vi "StatusTcpLink.vi"(0 "TCP Ref":refnum<k5>, 7 "VariableData":T1={"DecodeMode"="Stat", "LastSerial"=0, "NoReply"=FALSE, "StatCmd"="", "StatCmdReply"="", "StatCmdReplySerial"=0, "StatusPrefix"="", "StatusData"="", "SendOut"=FALSE, "StringCmd"=FALSE, "CmdString1"="", "CmdString0"="", "Astring1"=FALSE, "CmdDataOut"="", "CmdReply"="", "CmdReplySerial"=0, "CmdArray"=[0, 2, 1, 4, 16, 230, 2, 1, 0]}, 11 "error":errorcluster) -> (4 "TCP Ref":refnum<k5>, 8 "VariableData":T1={"DecodeMode"="Stat", "LastSerial"=0, "NoReply"=FALSE, "StatCmd"="", "StatCmdReply"="", "StatCmdReplySerial"=0, "StatusPrefix"="", "StatusData"="", "SendOut"=FALSE, "StringCmd"=FALSE, "CmdString1"="", "CmdString0"="", "Astring1"=FALSE, "CmdDataOut"="", "CmdReply"="", "CmdReplySerial"=0, "CmdArray"=[0, 2, 1, 4, 16, 230, 2, 1, 0]}, 15 "error out":errorcluster)   [LabVIEW 2020]
uses:
  TypeDefinitions/StatusVariableData.ctl
panel:
  out "Junk":string
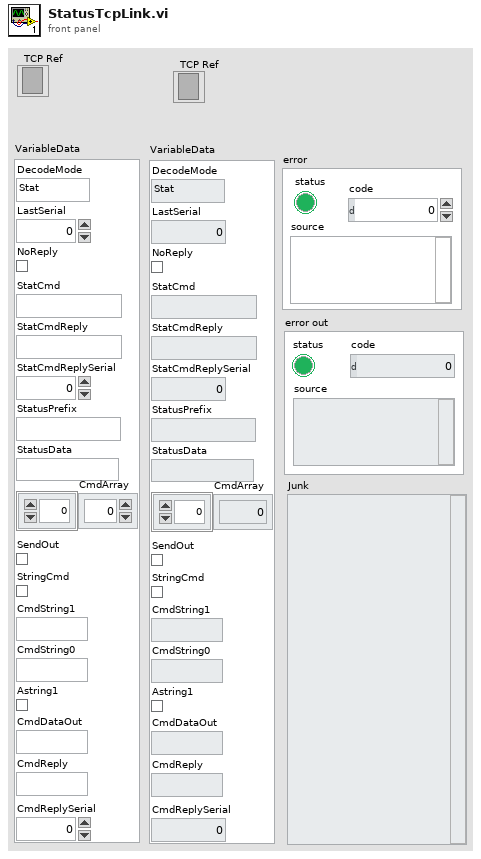
[diagram p1: front panel]
types:
  T1 = typedef "StatusVariableData.ctl" = cluster{"DecodeMode":string, "LastSerial":u32, "NoReply":bool, "StatCmd":string, "StatCmdReply":string, "StatCmdReplySerial":u32, "StatusPrefix":string, "StatusData":string, "SendOut":bool, "StringCmd":bool, "CmdString1":string, "CmdString0":string, "Astring1":bool, "CmdDataOut":string, "CmdReply":string, "CmdReplySerial":u32, "CmdArray":u32[]}
  T2 = enum16{"Standard", "Buffered", "CRLF", "Immediate"}
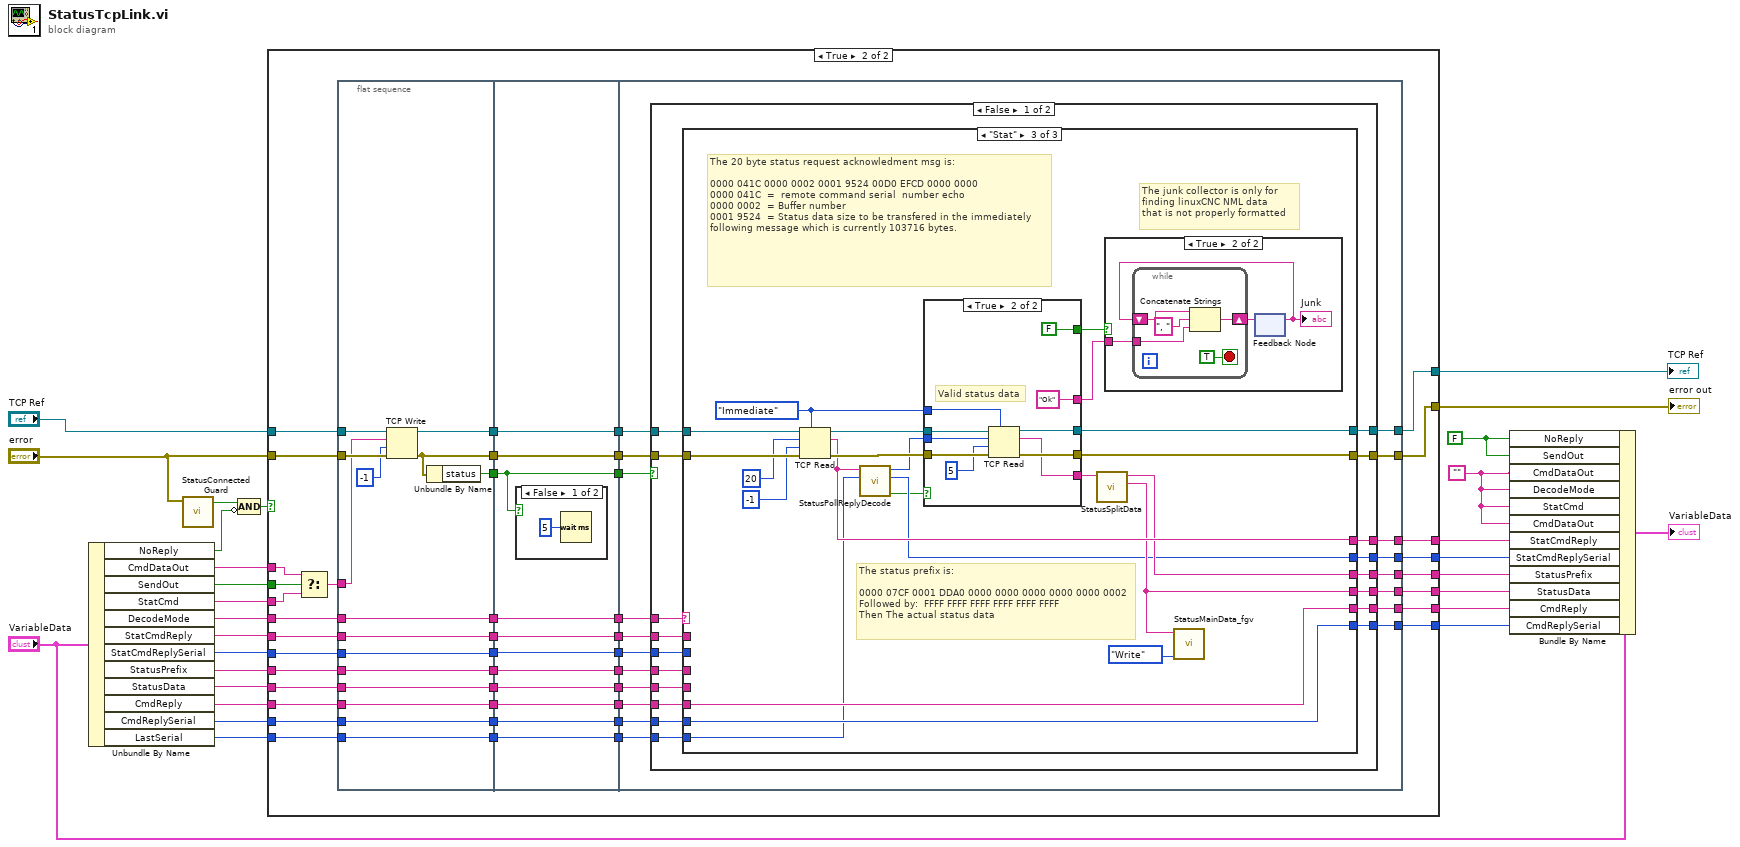
[diagram p0: block diagram]
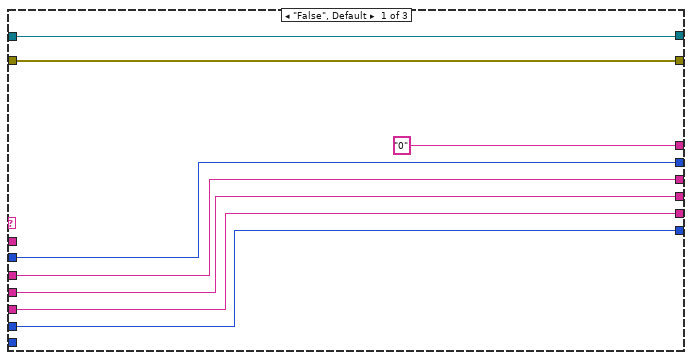
[diagram p4: hidden frame]
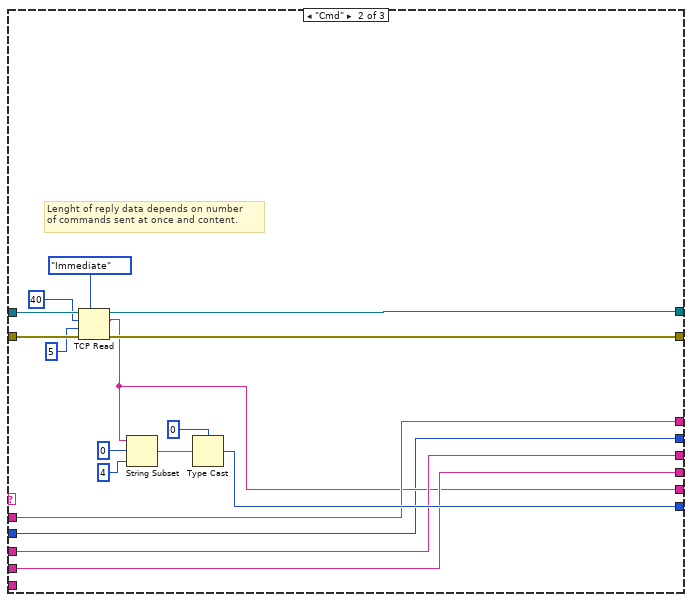
[diagram p5: hidden frame]
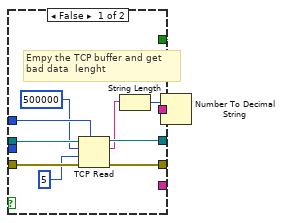
[diagram p7: hidden frame]
diagram:
  w2 = FALSE ("NoReply")
  w3 = ""
  n1 = Unbundle By Name("VariableData") -> ("NoReply"=w9:bool, "CmdDataOut"=w5:string, "SendOut"=w6:bool, "StatCmd"=w4:string, "DecodeMode"=w10:string, "StatCmdReply"=w11:string, "StatCmdReplySerial"=w12:u32, "StatusPrefix"=w13:string, "StatusData"=w14:string, "CmdReply"=w15:string, "CmdReplySerial"=w17:u32, "LastSerial"=w1:u32)
  n2 = call "StatusConnectedGuard.vi"("error"="error") -> ("EnableOut"=w8:bool)  [unwired: 10 in]
  n3 = Compound Arithmetic op=AND(w8, invert w9) -> (w7:bool)
  n4 = case shown="True" w7 {
    tunnel: "error" -> [w35 w72]
    tunnel: "TCP Ref" -> [w36 w71]
    tunnel: [w36 w70] -> w26
    tunnel: [w35 w44] -> w25
    tunnel: [w29 w57] -> w23
    tunnel: [w34 w56] -> w22
    tunnel: [w33 w55] -> w21
    tunnel: [w32 w54] -> w20
    tunnel: [w31 w53] -> w19
    tunnel: [w30 w52] -> w18
    tunnel: w17 -> [w30 w51]
    tunnel: w15 -> [w31 w50]
    tunnel: w14 -> [w32 w49]
    tunnel: w13 -> [w33 w48]
    tunnel: w12 -> [w34 w47]
    tunnel: w11 -> [w29 w46]
    tunnel: w10 -> [_ w45]
    tunnel: w6 -> [_ w43]
    tunnel: w5 -> [_ w42]
    tunnel: w4 -> [_ w41]
    tunnel: w1 -> [_ w39]
    frame False {
    }
    frame True {
      n5 = Select(t=w42, s=w43, f=w41) -> (s? t:f=w40:string)
      n6 = flat-sequence {
        tunnel: w45 -> [w95]
        tunnel: w71 -> [w92]
        tunnel: w72 -> [w90]
        tunnel: [w93] -> w80
        tunnel: [w91] -> w79
        tunnel: [w95] -> w78
        tunnel: [w94] -> w77
        tunnel: [w89] -> w68
        tunnel: w46 -> [w89]
        tunnel: [w85] -> w67
        tunnel: [w88] -> w64
        tunnel: w48 -> [w88]
        tunnel: w49 -> [w87]
        tunnel: [w87] -> w62
        tunnel: w50 -> [w86]
        tunnel: [w86] -> w60
        tunnel: [w84] -> w59
        tunnel: w47 -> [w85]
        tunnel: w51 -> [w84]
        tunnel: w40 -> [w83]
        tunnel: w39 -> [w81]
        tunnel: [w81] -> w38
        tunnel: [w104] -> w76
        tunnel: [w106] -> w75
        tunnel: [w105] -> w74
        tunnel: w80 -> [w104]
        tunnel: w79 -> [w106]
        tunnel: w78 -> [w105]
        tunnel: w77 -> [w103]
        tunnel: [w103] -> w73
        tunnel: [w102] -> w69
        tunnel: w68 -> [w102]
        tunnel: w67 -> [w101]
        tunnel: [w101] -> w66
        tunnel: [w100] -> w65
        tunnel: w64 -> [w100]
        tunnel: [w99] -> w63
        tunnel: w62 -> [w99]
        tunnel: [w98] -> w61
        tunnel: w60 -> [w98]
        tunnel: w59 -> [w97]
        tunnel: [w97] -> w58
        tunnel: w38 -> [w96]
        tunnel: [w96] -> w37
        tunnel: w76 -> [w126]
        tunnel: w75 -> [w125]
        tunnel: w74 -> [w124]
        tunnel: w73 -> [w123]
        tunnel: [w122] -> w54
        tunnel: [w121] -> w55
        tunnel: [w120] -> w57
        tunnel: [w119] -> w70
        tunnel: [w118] -> w44
        tunnel: [w117] -> w56
        tunnel: [w116] -> w53
        tunnel: [w115] -> w52
        tunnel: w69 -> [w114]
        tunnel: w66 -> [w113]
        tunnel: w65 -> [w112]
        tunnel: w63 -> [w111]
        tunnel: w61 -> [w110]
        tunnel: w58 -> [w109]
        tunnel: w37 -> [w108]
        frame #0 {
          n7 = TCP Write(connection ID=w92, data in=w83, error in (no error)=w90, 9:-1 ("timeout ms (25000)")) -> (connection ID out=w91:refnum<k5>, error out=w93:errorcluster)  [unwired: 1 out]
          n8 = Unbundle By Name(w93) -> ("status"=w94:bool)
        }
        frame #1 {
          n9 = case shown="False" w103 {
            frame False {
              n10 = Wait (ms)(milliseconds to wait=u32 5 ("millisecond multiple")) -> ()  [unwired: 1 out]
            }
            frame True {
            }
          }
        }
        frame #2 {
          n11 = case shown="False" w123 {
            tunnel: w126 -> [w144 w221]
            tunnel: w125 -> [w143 w222]
            tunnel: [w142 w222] -> w119
            tunnel: [w141 w221] -> w118
            tunnel: w124 -> [w140 _]
            tunnel: [w139 _] -> w122
            tunnel: [w138 _] -> w121
            tunnel: [w137 _] -> w120
            tunnel: [w136 _] -> w117
            tunnel: [w135 _] -> w116
            tunnel: [w134 _] -> w115
            tunnel: w114 -> [w133 _]
            tunnel: w113 -> [w132 _]
            tunnel: w112 -> [w131 _]
            tunnel: w111 -> [w130 _]
            tunnel: w110 -> [w129 _]
            tunnel: w109 -> [w128 _]
            tunnel: w108 -> [w127 _]
            frame False {
              n12 = case shown="\"Stat\"" w140 {
                tunnel: w143 -> [w151 w169 w182]
                tunnel: w144 -> [w152 w168 w190]
                tunnel: [w152 w155 w185] -> w141
                tunnel: [w151 w156 w186] -> w142
                tunnel: [w147 w158 w178] -> w139
                tunnel: [w148 w159 w179] -> w138
                tunnel: ["0" ("data out") w160 w183] -> w137
                tunnel: [w149 w153 w174] -> w136
                tunnel: [w146 w154 w189] -> w135
                tunnel: [w145 w161 w188] -> w134
                tunnel: w133 -> [_ w160 _]
                tunnel: w132 -> [w149 w153 _]
                tunnel: w131 -> [w148 w159 _]
                tunnel: w130 -> [w147 w158 _]
                tunnel: w129 -> [w146 _ w189]
                tunnel: w128 -> [w145 _ w188]
                tunnel: w127 -> [_ _ w171]
                frame "False", Default {
                }
                frame "Cmd" {
                  # "Lenght of reply data depends on number\nof commands sent at once and content."
                  n13 = TCP Read(connection ID=w169, bytes to read=40, error in (no error)=w168, 7:T2."Immediate" ("mode (standard)"), 9:5 ("timeout ms (25000)")) -> (connection ID out=w156:refnum<k5>, data out=w154:string, error out=w155:errorcluster)
                  n14 = String Subset(string=w154, offset (0)=0, length (rest)=4 ("length (rest)")) -> (substring=w164:string)
                  n15 = Type Cast(type=u32 0 ("y"), x=w164) -> (*(type *) &x=w161:u32)
                }
                frame "Stat" {
                  w170 = T2."Immediate" ("mode (standard)")
                  # "The junk collector is only for\nfinding linuxCNC NML data\nthat is not properly formatted"
                  # "The 20 byte status request acknowledment msg is:\n\n0000 041C 0000 0002 0001 9524 00D0 EFCD 0000 0000 \n0000 041C  =  remote command serial  number echo\n0000 0002  = Buffer number\n0001 9524  = Status data size to be transfered in the immediately\nfollowing message which is currently 103716 bytes."
                  # "The status prefix is:\n\n0000 07CF 0001 DDA0 0000 0000 0000 0000 0000 0002\nFollowed by:  FFFF FFFF FFFF FFFF FFFF FFFF \nThen The actual status data"
                  n16 = TCP Read(connection ID=w182, bytes to read=20, error in (no error)=w190, 7:w170, 9:-1 ("timeout ms (25000)")) -> (connection ID out=w187:refnum<k5>, data out=w183:string, error out=w184:errorcluster)
                  n17 = call "StatusPollReplyDecode.vi"("LastSerial"=w171, "data in"=w183) -> ("Boolean"=w172:bool, "SerialNumberEcho"=w174:u32, "StatusDataBytes"=w176:u32)  [unwired: 6 in, 1 out]
                  n18 = case shown="True" w172 {
                    tunnel: w187 -> [w207 w220]
                    tunnel: [w210 w219] -> w186
                    tunnel: [w209 w218] -> w185
                    tunnel: w184 -> [w208 w217]
                    tunnel: w170 -> [w206 w216]
                    tunnel: [_ w215] -> w177
                    tunnel: w176 -> [_ w213]
                    tunnel: [w201 "Ok"] -> w175
                    tunnel: [TRUE FALSE] -> w173
                    frame False {
                      # "Empy the TCP buffer and get\nbad data  lenght"
                      n19 = TCP Read(connection ID=w207, bytes to read=500000, error in (no error)=w208, 7:w206, 9:5 ("timeout ms (25000)")) -> (connection ID out=w210:refnum<k5>, data out=w202:string, error out=w209:errorcluster)
                      n20 = String Length(string=w202) -> (length=w203:i32)
                      n21 = Number To Decimal String(number=w203) -> (decimal integer string=w201:string)  [unwired: 1 in]
                    }
                    frame True {
                      # "Valid status data"
                      n22 = TCP Read(connection ID=w220, bytes to read=w213, error in (no error)=w217, 7:w216, 9:5 ("timeout ms (25000)")) -> (connection ID out=w219:refnum<k5>, data out=w215:string, error out=w218:errorcluster)
                    }
                  }
                  n23 = call "StatusSplitData.vi"("StatusData in"=w177) -> ("StatusData out"=w178:string, "StatusPrefix"=w179:string)  [unwired: 9 in]
                  n24 = case shown="True" w173 {
                    tunnel: w175 -> [_ w192]
                    frame False {
                    }
                    frame True {
                      n25 = feedback #1() -> (w194:string)  [unwired: 1 in]
                      "Junk" <- w194
                      n26 = while {
                        shift-right: [w198] -> w193
                        shift-left: w194 -> [w197]
                        tunnel: w192 -> [w196]
                        stop <- TRUE stop-if-true
                        n27 = Concatenate Strings(w197, ", ", w196) -> (w198:string)
                      }
                      n28 = feedback-in #1(w193) -> ()
                    }
                  }
                  n29 = call "StatusMainData_fgv.vi"("Enum"=enum16{"Read", "Write"}."Write", "StatusData"=w178) -> ()  [unwired: 9 in, 1 out]
                }
              }
            }
            frame True {
            }
          }
        }
      }
    }
  }
  "error out" <- w25
  "TCP Ref" <- w26
  n30 = Bundle By Name(cluster="VariableData", "NoReply"=w2, "SendOut"=w2, "CmdDataOut"=w3, "DecodeMode"=w3, "StatCmd"=w3, "CmdDataOut"=w3, "StatCmdReply"=w23, "StatCmdReplySerial"=w22, "StatusPrefix"=w21, "StatusData"=w20, "CmdReply"=w19, "CmdReplySerial"=w18) -> (→"VariableData":T1)
